vi "Servo MSMT Set RF Power.vi"(8 "error in (no error)":errorcluster, 10 "Step In":refnum<k7>, 11 "Servo MSMT in":refnum<class "Servo MSMT.lvclass">) -> (0 "error out":errorcluster, 2 "Step Out":refnum<k7>, 3 "Servo MSMT out":refnum<class "Servo MSMT.lvclass">)   [LabVIEW 2018, in "Servo MSMT.lvlib" / "Servo MSMT.lvclass"]
uses:
  Servo MSMT.lvclass
  C:/Sequence Automation/Plugins/Measurement Interface.lvlibp/Measurement Interface.lvclass
  Plugins/Measurement Interface.lvlibp/Public Methods/Sequence Reference/Read Sequence Reference.vi
  Plugins/Measurement Interface.lvlibp/Private Methods/Measurement Name/Read Measurement Name.vi
  Plugins/TestStand API Tools (TSAT).lvlibp/Sequence Actions/TSAT Sequence Actions.lvlib
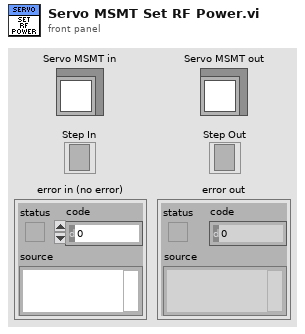
[diagram p1: front panel]
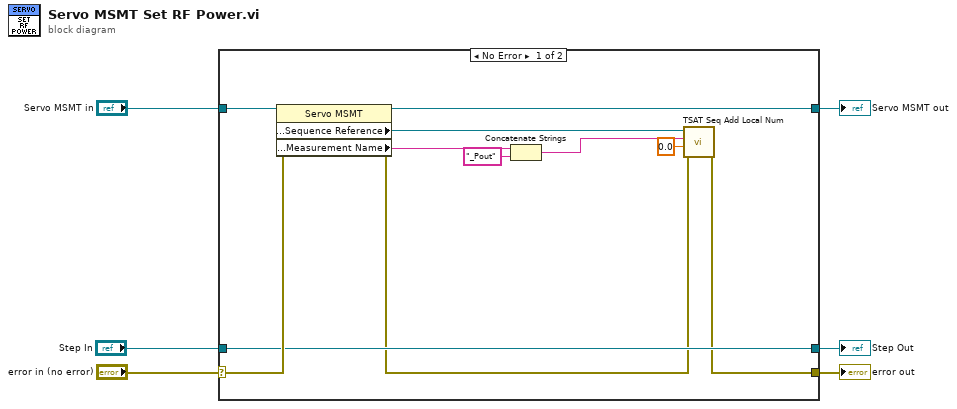
[diagram p0: block diagram]
diagram:
  n1 = case shown="No Error" "error in (no error)" {
    selector: "error in (no error)" -> [w17 w20]
    tunnel: [w11 w20] -> w5
    tunnel: [w14 w19] -> w3
    tunnel: "Servo MSMT in" -> [w15 w19]
    tunnel: "Step In" -> [w16 w18]
    tunnel: [w16 w18] -> w1
    frame No Error {
      n2 = property class="Servo MSMT"(reference=w15, error in=w17) -> (reference out=w14:refnum<class "Servo MSMT.lvclass">, error out=w12:errorcluster, "Public Methods:Sequence Reference"=w13:refnum<k7>, "Public Methods:Measurement Name"=w10:string)
      n3 = Concatenate Strings(w10, "_Pout" ("string")) -> (w8:string)
      n4 = call "TSAT Seq Add Local Num.vi"("Error In"=w12, "Variable Value"=0.0, "Local Variable Name"=w8, "Sequence In"=w13) -> ("Error Out"=w11:errorcluster)  [unwired: 6 in, 1 out]
    }
    frame Error {
    }
  }
  "error out" <- w5
  "Servo MSMT out" <- w3
  "Step Out" <- w1
